vi "Rcv Caller Content.vi"(8 "error in (no error)":errorcluster, 10 "Content":string, 11 "Nested Actor in":refnum<class "Nested Actor.lvclass">) -> (0 "error out":errorcluster, 3 "Nested Actor out":refnum<class "Nested Actor.lvclass">)   [LabVIEW 2020, in "Nested Actor.lvlib" / "Nested Actor.lvclass"]
uses:
  Nested Actor.lvclass
  Nested Actor.lvclass/Nested Actor.ctl
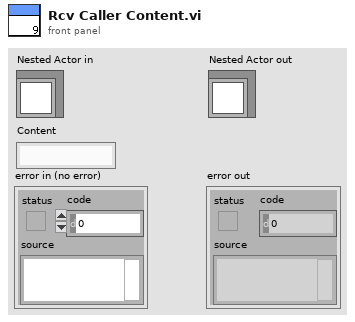
[diagram p1: front panel]
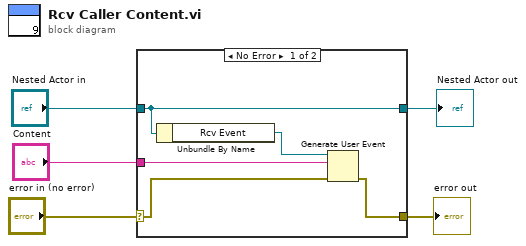
[diagram p0: block diagram]
diagram:
  n1 = case shown="No Error" "error in (no error)" {
    selector: "error in (no error)" -> [w7 w12]
    tunnel: [w6 w12] -> w4
    tunnel: [w10 w11] -> w2
    tunnel: "Nested Actor in" -> [w10 w11]
    tunnel: "Content" -> [w8 _]
    frame No Error {
      n2 = Unbundle By Name(w10) -> ("Rcv Event"=w9:refnum<user-event>)
      n3 = Generate User Event(user event=w9, event data cluster=w8, error in=w7) -> (error out=w6:errorcluster)  [unwired: 1 in, 1 out]
    }
    frame Error {
    }
  }
  "error out" <- w4
  "Nested Actor out" <- w2
